vi "NI myRIO Post-Install App Launcher.vi"(10 "Variant":variant) -> (0 "error out":errorcluster)   [LabVIEW 2013]
uses:
  <resource>/dialog/NewProjectWizard/NewProjectDialogCallingModes.ctl
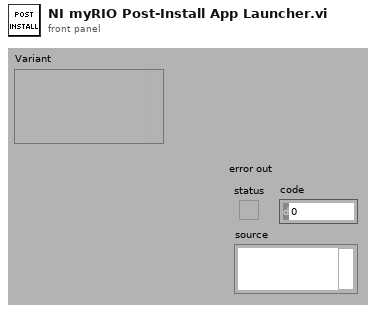
[diagram p1: front panel]
types:
  T1 = typedef "NewProjectDialogCallingModes.ctl" = enum16{"Default", "Open to 2nd Page", "Open Recent Item"}
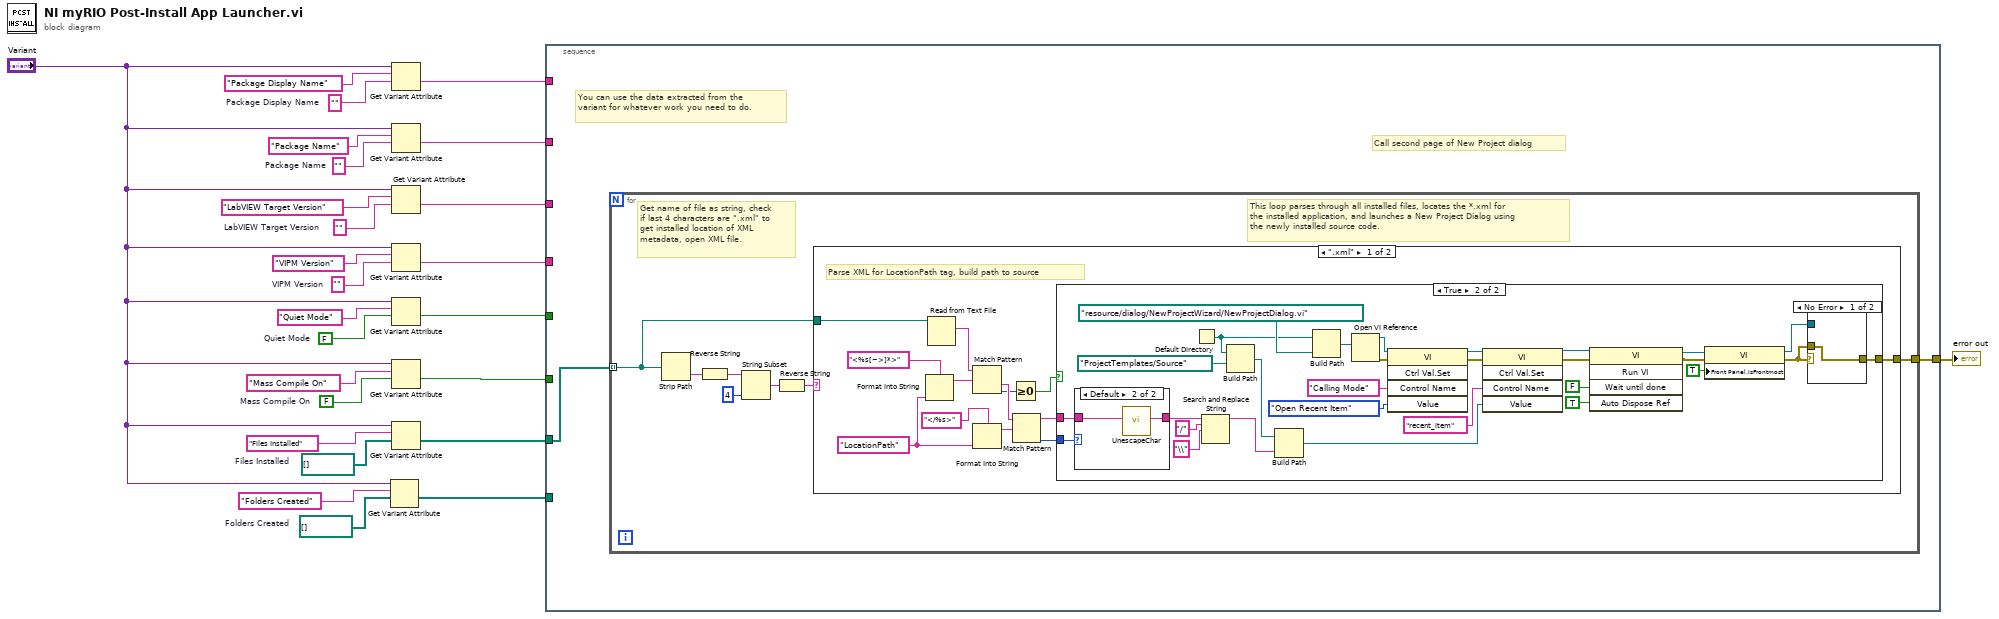
[diagram p0: block diagram]
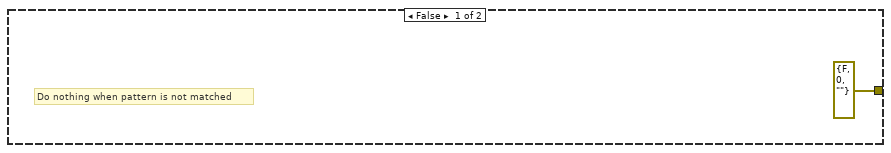
[diagram p2: hidden frame]
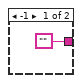
[diagram p3: hidden frame]
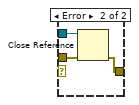
[diagram p4: hidden frame]
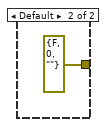
[diagram p5: hidden frame]
diagram:
  w2 = path[] []  # Folders Created
  w3 = path[] []  # Files Installed
  w9 = FALSE  # Mass Compile On
  w10 = ""  # Package Display Name
  w17 = FALSE  # Quiet Mode
  w20 = ""  # VIPM Version
  w22 = ""  # LabVIEW Target Version
  w24 = ""  # Package Name
  n1 = Get Variant Attribute(Variant="Variant", name="Folders Created", default value (empty Variant)=w2) -> (value=w7:path[])  [unwired: 1 in, 3 out]
  n2 = Get Variant Attribute(Variant="Variant", name="Package Display Name", default value (empty Variant)=w10) -> (value=w16:string)  [unwired: 1 in, 3 out]
  n3 = Get Variant Attribute(Variant="Variant", name="Package Name", default value (empty Variant)=w24) -> (value=w15:string)  [unwired: 1 in, 3 out]
  n4 = Get Variant Attribute(Variant="Variant", name="LabVIEW Target Version", default value (empty Variant)=w22) -> (value=w14:string)  [unwired: 1 in, 3 out]
  n5 = Get Variant Attribute(Variant="Variant", name="VIPM Version", default value (empty Variant)=w20) -> (value=w13:string)  [unwired: 1 in, 3 out]
  n6 = Get Variant Attribute(Variant="Variant", name="Quiet Mode", default value (empty Variant)=w17) -> (value=w12:bool)  [unwired: 1 in, 3 out]
  n7 = Get Variant Attribute(Variant="Variant", name="Mass Compile On", default value (empty Variant)=w9) -> (value=w11:bool)  [unwired: 1 in, 3 out]
  n8 = Get Variant Attribute(Variant="Variant", name="Files Installed", default value (empty Variant)=w3) -> (value=w6:path[])  [unwired: 1 in, 3 out]
  n9 = stacked-sequence {
    tunnel: w16 -> [_]
    tunnel: w15 -> [_]
    tunnel: w14 -> [_]
    tunnel: w13 -> [_]
    tunnel: w12 -> [_]
    tunnel: w11 -> [_]
    tunnel: w6 -> [w28]
    tunnel: w7 -> [_]
    tunnel: [w27] -> w1
    frame #0 {
      # "Call second page of New Project dialog"
      # "You can use the data extracted from the variant for whatever work you need to do."
      n10 = for {
        tunnel: w28 -> [w29] mode=indexing
        tunnel: [w35] -> w27
        # "This loop parses through all installed files, locates the *.xml for \nthe installed application, and launches a New Project Dialog using\nthe newly installed source code."
        # "Get name of file as string, check\nif last 4 characters are \".xml\" to \nget installed location of XML\nmetadata, open XML file."
        n11 = Strip Path(path=w29) -> (name=w34:string)  [unwired: 1 out]
        n12 = Reverse String(1:w34) -> (0:w33:string)
        n13 = String Subset(string=w33, length (rest)=4 ("length (rest)")) -> (substring=w31:string)  [unwired: 1 in]
        n14 = Reverse String(1:w31) -> (0:w30:string)
        n15 = case shown="\".xml\"" w30 {
          tunnel: [w48 errorcluster {"status"=FALSE, "code"=0, "source"=""} ("error out")] -> w35
          tunnel: w29 -> [w37 _]
          frame ".xml" {
            w44 = "LocationPath" ("tag")
            # "Parse XML for LocationPath tag, build path to source"
            n16 = Format Into String(format string="<%s[~>]*>" ("regular expression"), w44) -> (resulting string=w43:string)  [unwired: 2 in, 1 out]
            n17 = Read from Text File(file (use dialog)=w37) -> (text=w38:string)  [unwired: 3 in, 3 out]
            n18 = Match Pattern(string=w38, regular expression=w43) -> (after substring=w47:string, offset past match=w40:i32)  [unwired: 1 in, 2 out]
            n19 = Format Into String(format string="</%s>" ("regular expression"), w44) -> (resulting string=w42:string)  [unwired: 2 in, 1 out]
            n20 = Greater Or Equal To 0?(x=w40) -> (x >= 0?=w36:bool)
            n21 = Match Pattern(string=w47, regular expression=w42) -> (before substring=w41:string, offset past match=w39:i32)  [unwired: 1 in, 2 out]
            n22 = case shown="True" w36 {
              tunnel: [errorcluster {"status"=FALSE, "code"=0, "source"=""} ("error out") w71] -> w48
              tunnel: w41 -> [_ w64]
              tunnel: w39 -> [_ w63]
              frame False {
                # "Do nothing when pattern is not matched"
              }
              frame True {
                n23 = case shown="Default" w63 {
                  tunnel: w64 -> [_ w81]
                  tunnel: ["" w80] -> w61
                  frame -1 {
                  }
                  frame Default {
                    n24 = call <vilib>:"UnescapeChar.vi"("XML In"=w81) -> ("XML Out"=w80:string)  [unwired: 10 in]
                  }
                }
                n25 = Default Directory() -> (w57:path)
                n26 = Search and Replace String(input string=w61, search string="/", replace string="\\" ("replace string (\"\")")) -> (result string=w60:string)  [unwired: 5 in, 3 out]
                n27 = Build Path(base path=w57, name or relative path=path "ProjectTemplates/Source") -> (appended path=w62:path)
                n28 = Build Path(base path=w62, name or relative path=w60) -> (appended path=w55:path)
                n29 = Build Path(base path=w57, name or relative path=path "resource/dialog/NewProjectWizard/NewProjectDialog.vi") -> (appended path=w73:path)
                n30 = Open VI Reference(vi path=w73) -> (vi reference=w70:refnum<vi>, error out=w69:errorcluster)  [unwired: 5 in]
                n31 = invoke class="VI" method="Ctrl Val.Set"(reference=w70, error in=w69, "Control Name"="Calling Mode", "Value"=NewProjectDialogCallingModes."Open Recent Item" ("Calling Mode")) -> (reference out=w77:refnum<vi>, error out=w78:errorcluster)  [unwired: 1 in, 3 out]
                n32 = invoke class="VI" method="Ctrl Val.Set"(reference=w77, error in=w78, "Control Name"="recent_item", "Value"=w55) -> (reference out=w66:refnum<vi>, error out=w65:errorcluster)  [unwired: 1 in, 3 out]
                n33 = invoke class="VI" method="Run VI"(reference=w66, error in=w65, "Wait until done"=FALSE ("Wait Until Done"), "Auto Dispose Ref"=TRUE ("Auto Dispose Reference")) -> (reference out=w54:refnum<vi>, error out=w53:errorcluster)  [unwired: 1 in, 3 out]
                n34 = property class="VI"(reference=w54, error in=w53, "Front Panel.IsFrontmost"=TRUE ("Front Panel Window:Is Frontmost")) -> (reference out=w50:refnum<vi>, error out=w52:errorcluster)
                n35 = case shown="No Error" w52 {
                  tunnel: w50 -> [_ w85]
                  tunnel: w52 -> [w82 w84]
                  tunnel: [w82 w83] -> w71
                  frame No Error {
                  }
                  frame Error {
                    n36 = Close Reference(reference=w85, error in (no error)=w84) -> (error out=w83:errorcluster)
                  }
                }
              }
            }
          }
          frame Default {
          }
        }
      }
    }
  }
  "error out" <- w1
